vi "Flash Title Bar.vi"(7 "flash time":u32=100 caption="flash time (ms) (100)", 8 "error in":errorcluster caption="error in (no error)" {"code" format="%d\n%x"}, 9 "number of flashes (1)":i32=1, 10 "window name (\"\")":string, 11 "window refnum":T1 caption="window refnum (NaWR)") -> (0 "error out":errorcluster {"code" format="%d\n%x"}, 3 "window refnum out":T1)   [LabVIEW 2020, in "Win Util New.lvlib"]
doc: "This function will make the title bar of the window named in the 'window name' input, or identified by the 'window refnum' flash once, the state of the title bar changing at the specified rate the given number of times. If 'not a window refnum' is passed in, then the function will use the window name to get a window window refnum. If the window cannot be found, an error will be returned."
uses:
  Win Util New.lvlib
  Window Refnum.ctl
  user32.dll
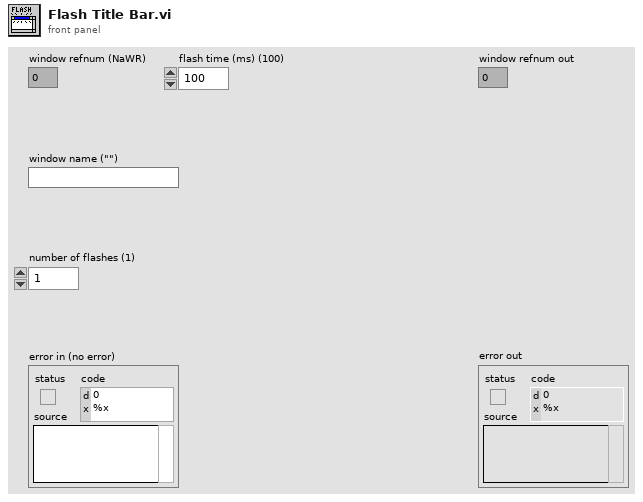
[diagram p1: front panel]
types:
  T1 = typedef "Win Util New.lvlib/Window Refnum.ctl" = u64
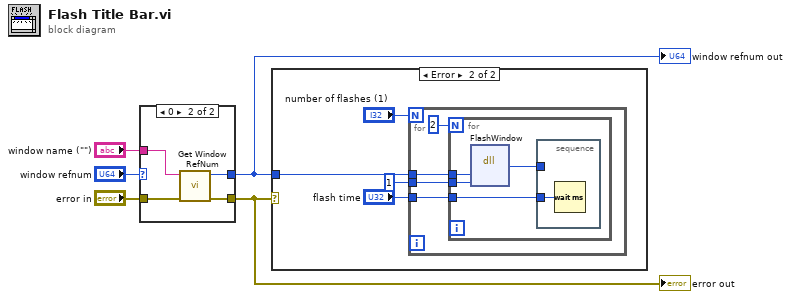
[diagram p0: block diagram]
diagram:
  n1 = case shown="0" "window refnum" {
    selector: "window refnum" -> [w6 _]
    tunnel: "error in" -> [w7 w11]
    tunnel: [w6 w10] -> w5
    tunnel: [w7 w9] -> w1
    tunnel: "window name (\"\")" -> [_ w8]
    frame Default {
    }
    frame 0 {
      n2 = call "Get Window RefNum.vi"("error in"=w11, "window name (\"\")"=w8) -> ("error out"=w9:errorcluster, "window refnum (NaWR)"=w10:T1)  [unwired: 6 out]
    }
  }
  "error out" <- w1
  "window refnum out" <- w5
  n3 = case shown="Error" w1 {
    tunnel: w5 -> [_ w12]
    frame No Error {
    }
    frame Error {
      n4 = for {
        N: "number of flashes (1)" -> [_]
        tunnel: "flash time" -> [w18]
        tunnel: 1 -> [w17]
        tunnel: w12 -> [w16]
        n5 = for {
          N: 2 -> [_]
          tunnel: w18 -> [w23]
          tunnel: w17 -> [w22]
          tunnel: w16 -> [w21]
          n6 = dll-call lib="USER32.DLL" fn="FlashWindow"("hWnd"=w21, "fInvert"=w22) -> ("active?"=w20:i32)  [unwired: 5 in, 2 out]
          n7 = stacked-sequence {
            tunnel: w23 -> [w24]
            tunnel: w20 -> [_]
            frame #0 {
              n8 = Wait (ms)(milliseconds to wait=w24) -> ()  [unwired: 1 out]
            }
          }
        }
      }
    }
  }
